vi "Remove empty Errors.vi"(7 "Remove Warnings(true)":bool=TRUE, 8 "all error clusters":errorcluster[](array[cluster])) -> (0 "err and warnings":errorcluster[](array[cluster]), 2 "some problems?":bool)   [LabVIEW 2009, in "POLARIS BME DG.lvlib"]
doc: "Gets a array with LV error clusters and removes elements containing no error. If You want keep warnings set \"Remove Warnings\" = false. If array contains no elements with errors, output \"some problems?\" is false\n\n------------------\n\nauthor: Alexander Kessler, Helmholtz-Institut-Jena \nmaintainer: Alexander Kessler: alexander.kessler@uni-jena.de\n\nLicense Agreement for this software:\n\nCopyright (C)\nHelmholtz-Institut-Jena\nFröbelsteg 3\n07743 Jena\nGermany\n\nContact: alexander.kessler@uni-jena.de\n\nThis program is free software; you can redistribute it and/or modify it under the terms of the GNU General Public License as published by the Free Software Foundation; either version 2 of the license, or (at your option) any later version.\n\nThis program is distributed in the hope that it will be useful, but WITHOUT ANY WARRANTY; without even the implied warranty of MERCHANTABILITY or FITNESS FOR A PARTICULAR PURPOSE. See the GNU General License for more details (http://www.gnu.org)."
uses:
  POLARIS BME DG.lvlib
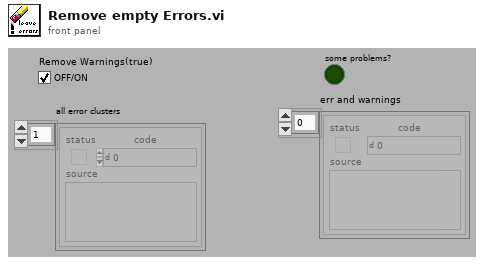
[diagram p1: front panel]
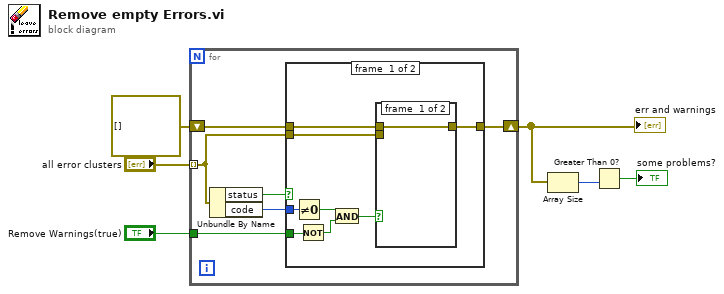
[diagram p0: block diagram]
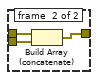
[diagram p2: hidden frame]
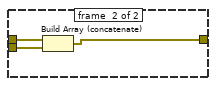
[diagram p3: hidden frame]
diagram:
  n1 = for {
    tunnel: "all error clusters" -> [w11] mode=indexing
    tunnel: "Remove Warnings(true)" -> [w7]
    shift-right: [w10] -> w3
    shift-left: errorcluster[] [] -> [w9]
    n2 = Unbundle By Name(w11) -> ("status"=w12:bool, "code"=w8:i32)
    n3 = case shown="False" w12 {
      tunnel: w11 -> [w14 w27]
      tunnel: [w13 w26] -> w10
      tunnel: w9 -> [w15 w25]
      tunnel: w8 -> [w20 _]
      tunnel: w7 -> [w18 _]
      frame #0 {
        n4 = Not Equal To 0?(x=w20) -> (x != 0?=w19:bool)
        n5 = Not(x=w18) -> (.not. x?=w17:bool)
        n6 = And(x=w19, y=w17) -> (x .and. y?=w16:bool)
        n7 = case shown="False" w16 {
          tunnel: w15 -> [w21 w24]
          tunnel: w14 -> [_ w23]
          tunnel: [w21 w22] -> w13
          frame #0 {
          }
          frame #1 {
            n8 = Build Array (concatenate)(w24, w23) -> (w22:errorcluster[])
          }
        }
      }
      frame #1 {
        n9 = Build Array (concatenate)(w25, w27) -> (w26:errorcluster[])
      }
    }
  }
  "err and warnings" <- w3
  n10 = Array Size(array=w3) -> (size(s)=w2:i32)
  n11 = Greater Than 0?(x=w2) -> (x > 0?=→"some problems?":bool)
